vi "new FGGA Serial Data Server & Recordingv5.0_10Hz_Scroll_Pump.vi"(0 "VISA resource name out":refnum<visa-resource-name>, 11 "error IO":errorcluster) -> ()   [LabVIEW 2014]
uses:
  <vilib>/Platform/TimedLoop/XDataNode/timing_clust.ctl
  <vilib>/Platform/TimedLoop/XDataNode/nitl_modes.ctl
  <vilib>/Platform/TimedLoop/XDataNode/wakeup.ctl
  C:/Program Files (x86)/National Instruments/LabVIEW 2014/examples/Data Communication/Network Streams/Simple Network Streams/support/Network Stream Command.ctl
  <vilib>/Utility/error.llb/whitespace.ctl
  <vilib>/Instr/_visa.llb/VISA Flush IO Buffer Mask.ctl
  <vilib>/Instr/_visa.llb/VISA Configure Serial Port (Instr).vi
  <vilib>/Utility/tcp.llb/UDP Multicast Write-Only Open.vi
  <vilib>/platform/TimedLoop/XDataNode/XDataNode.xnode
  <vilib>/Platform/TimedLoop/XDataNode/XDNodeRunTimeDep.lvlib
panel:
  out "V12":bool
  out "V11":bool
  out "V10":bool
  out "FLOW ALL OFF":bool
  out "LOW FLOW MASTER SWITCH":bool
  out "HIGH FLOW MASTER SWITCH":bool
  out "ASCII_file_out":string
  out "Unix time":u32
  out "FGGA Pump":bool
  out "Flight Number":string
  out "Stop File Write":bool
  out "Default file name":string
  out "MFC":dbl[](array[numeric])
  out "FGGA restart":bool
  out "V4":bool
  out "V3":bool
  out "V2":bool
  out "V1":bool
  out "error out 2":errorcluster
  out "error out":errorcluster
  in  "MFC_1 SLPM set value":dbl
  out "Value Read":string
  out "status":bool
  in  "VISA resource name":refnum<visa-resource-name>="ASRL3::INSTR"
  in  "timeout (10sec) 2":u32=3000
  in  "Clear Display\nErrors":bool
  out "Data Processing":bool
  out "TCP Binary Packet":string
  out "UDP Time Stamp Offset":i32=1
  out "Data String":string
  out "UDP_ACSII_Out":string
  out "Serial error out":errorcluster
  out "SEPTIC TCP Error Out":errorcluster
  out "TCP packet\nSend To SEPTIC":bool
  out "FISH TCP Error Out":errorcluster
  out "TCP packet\nSend To FISH":bool
  out "UDP_Pack_num":u32
  out "UDP_Out Status":bool
  out "UDP_Out_Error Out":errorcluster
  out "Data Array":string[](array[string])
  out "RAW DATA":string
  in  "stop":bool
  out "Number of times \nRead time out":u32
  out "Loop count":i32
  # "Date"
  # "Time"
  # "CH4_wet_ppm"
  # "1"
  # "H2O_ppm"
  # "CO2_wet_ppm"
  # "CH4_dry_ppm"
  # "CO2_dry_ppm"
  # "cell_pressure_torr"
  # "cell_temp_degC"
  # "ambient(bench)_temp_degC"
  # "RDA_us"
  # "RDB_us"
  # "Fitflag"
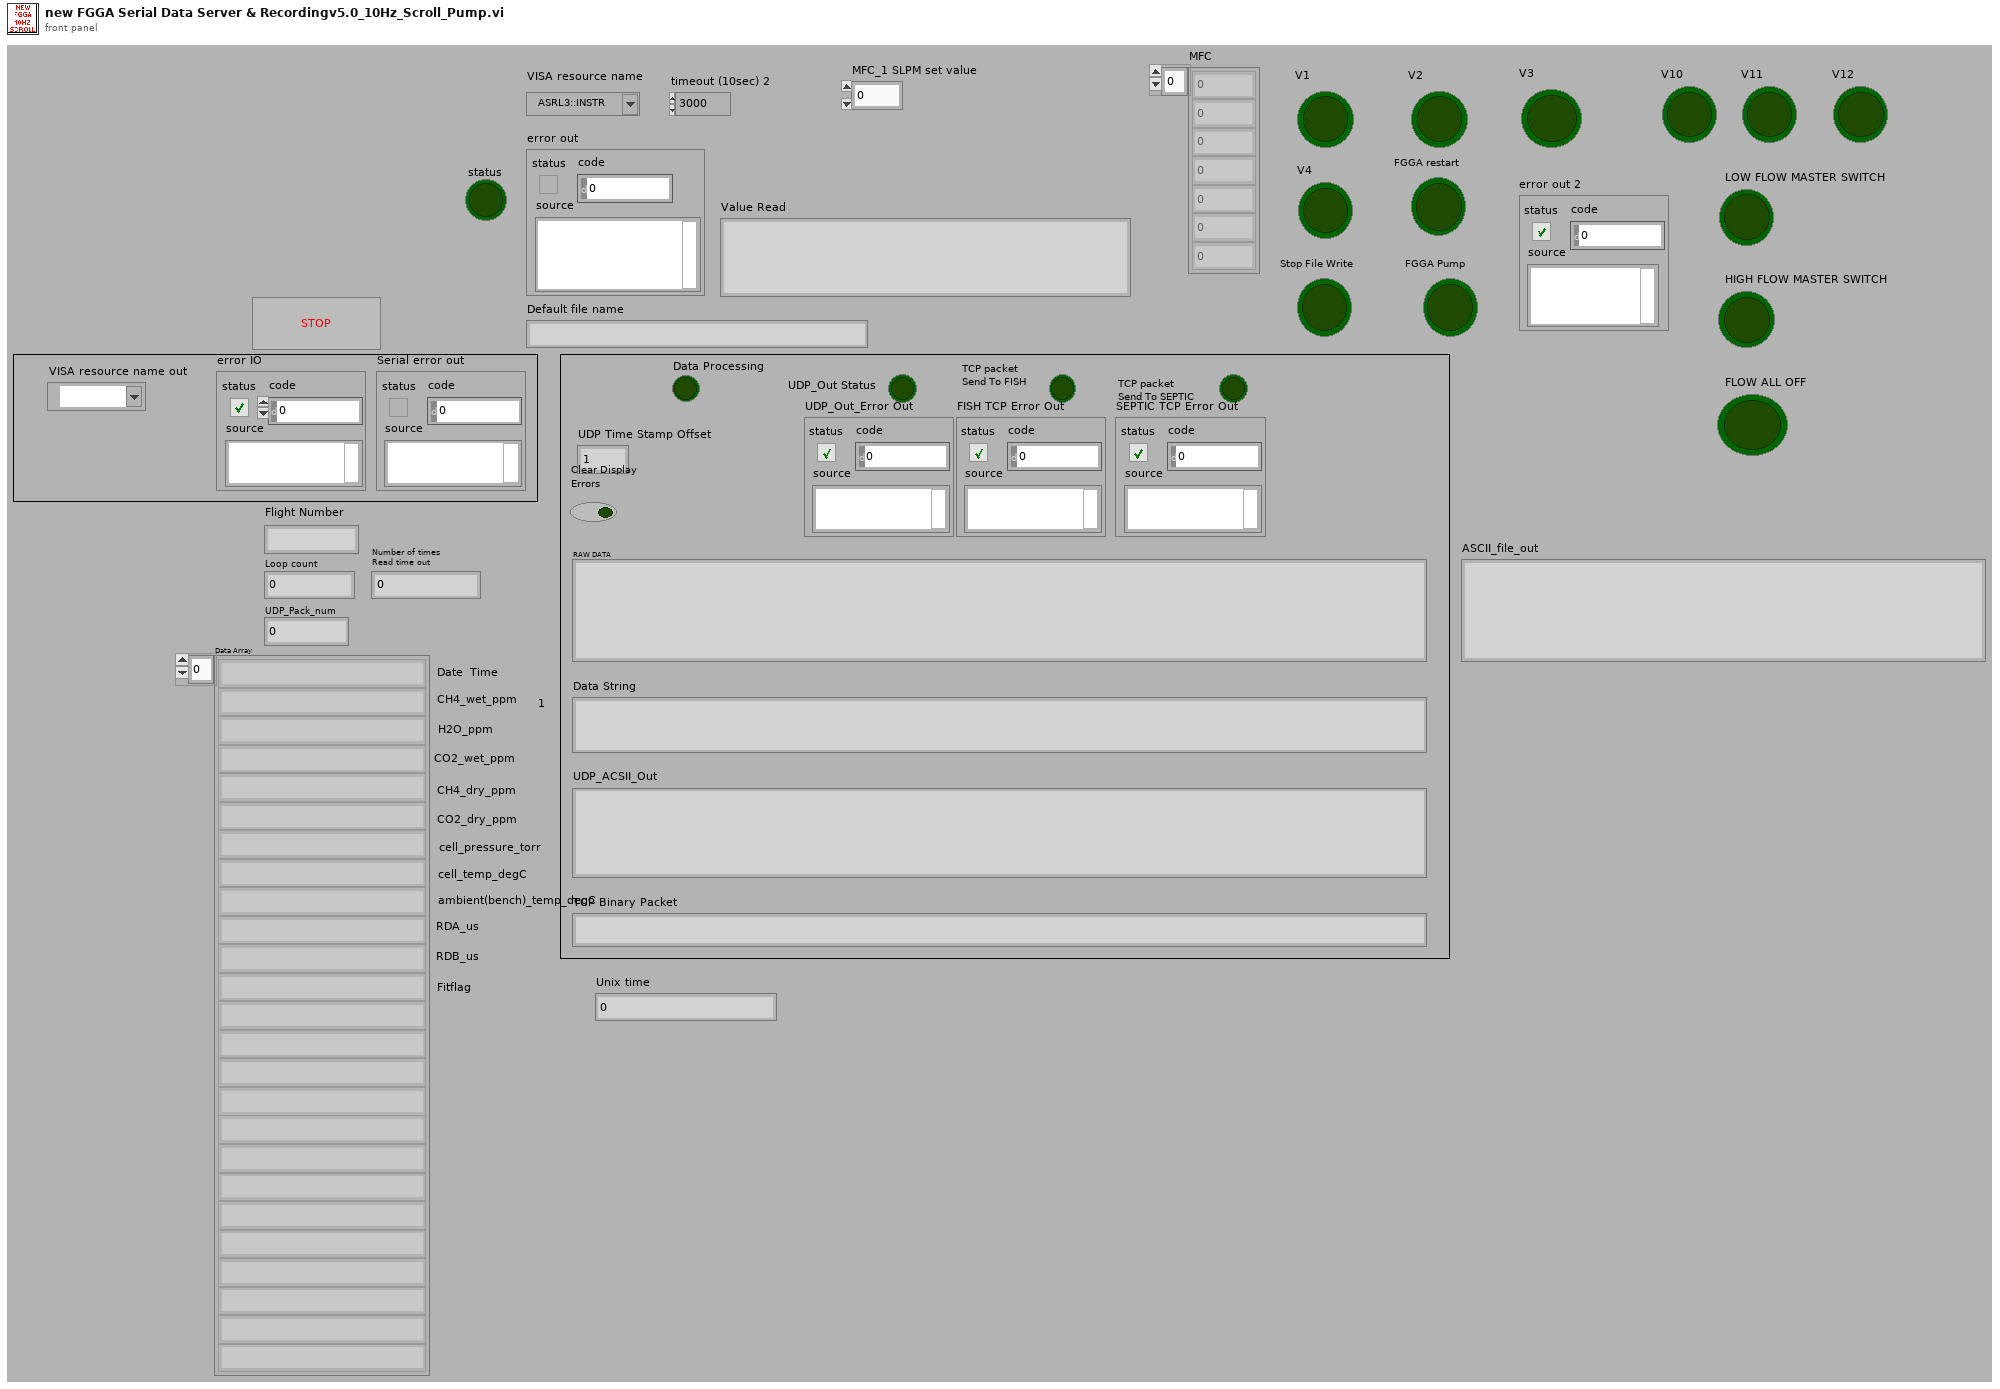
[diagram p1: front panel]
types:
  T1 = typedef "XDNodeRunTimeDep.lvlib/timing_clust.ctl" = cluster{"Expected End [f-1]":u64, "Actual End [f-1]":u64, "Finished Late? [f-1]":bool, "Expected End [i-1]":u64, "Actual End [i-1]":u64, "Finished Late? [i-1]":bool, "Expected Start [i]":u64, "Actual Start [i]":u64, "Expected Start [f]":u64, "Actual Start [f]":u64, "Source Name":string, "Structure Name":string, "Period":i64, "Deadline":i64, "Offset":i64, "Start":i64, "Priority":i32, "Timeout":i32, "Mode":T2, "Wakeup Reason":T3, "Error":errorcluster, "Source Type":string, "Secondary Source Type":string, "Global End Time":u64, "Global Start Time":u64, "Frame Duration":u64, "Iteration Duration":u64, "Assigned CPU":i32, "I/O Scan Engine Mode":u32}
  T2 = typedef "XDNodeRunTimeDep.lvlib/nitl_modes.ctl" = enum32{"No Change", "Process missed periods, maintain original phase", "Discard missed periods, maintain original phase", "Process missed periods, ignore original phase", "Discard missed periods, ignore original phase"}
  T3 = typedef "XDNodeRunTimeDep.lvlib/wakeup.ctl" = enum32{"Normal", "Aborted", "Asynchronous wakeup", "Timing source error", "Timed loop error", "Timeout"}
  T4 = enum16{"open", "replace", "create", "open or create", "replace or create", "replace or create with confirmation"}
  T5 = typedef "Network Stream Command.ctl" = cluster{"Message":string, "Message Data":variant}
  T6 = typedef "whitespace.ctl" = u16
  T7 = typedef "VISA Flush IO Buffer Mask.ctl" = u16
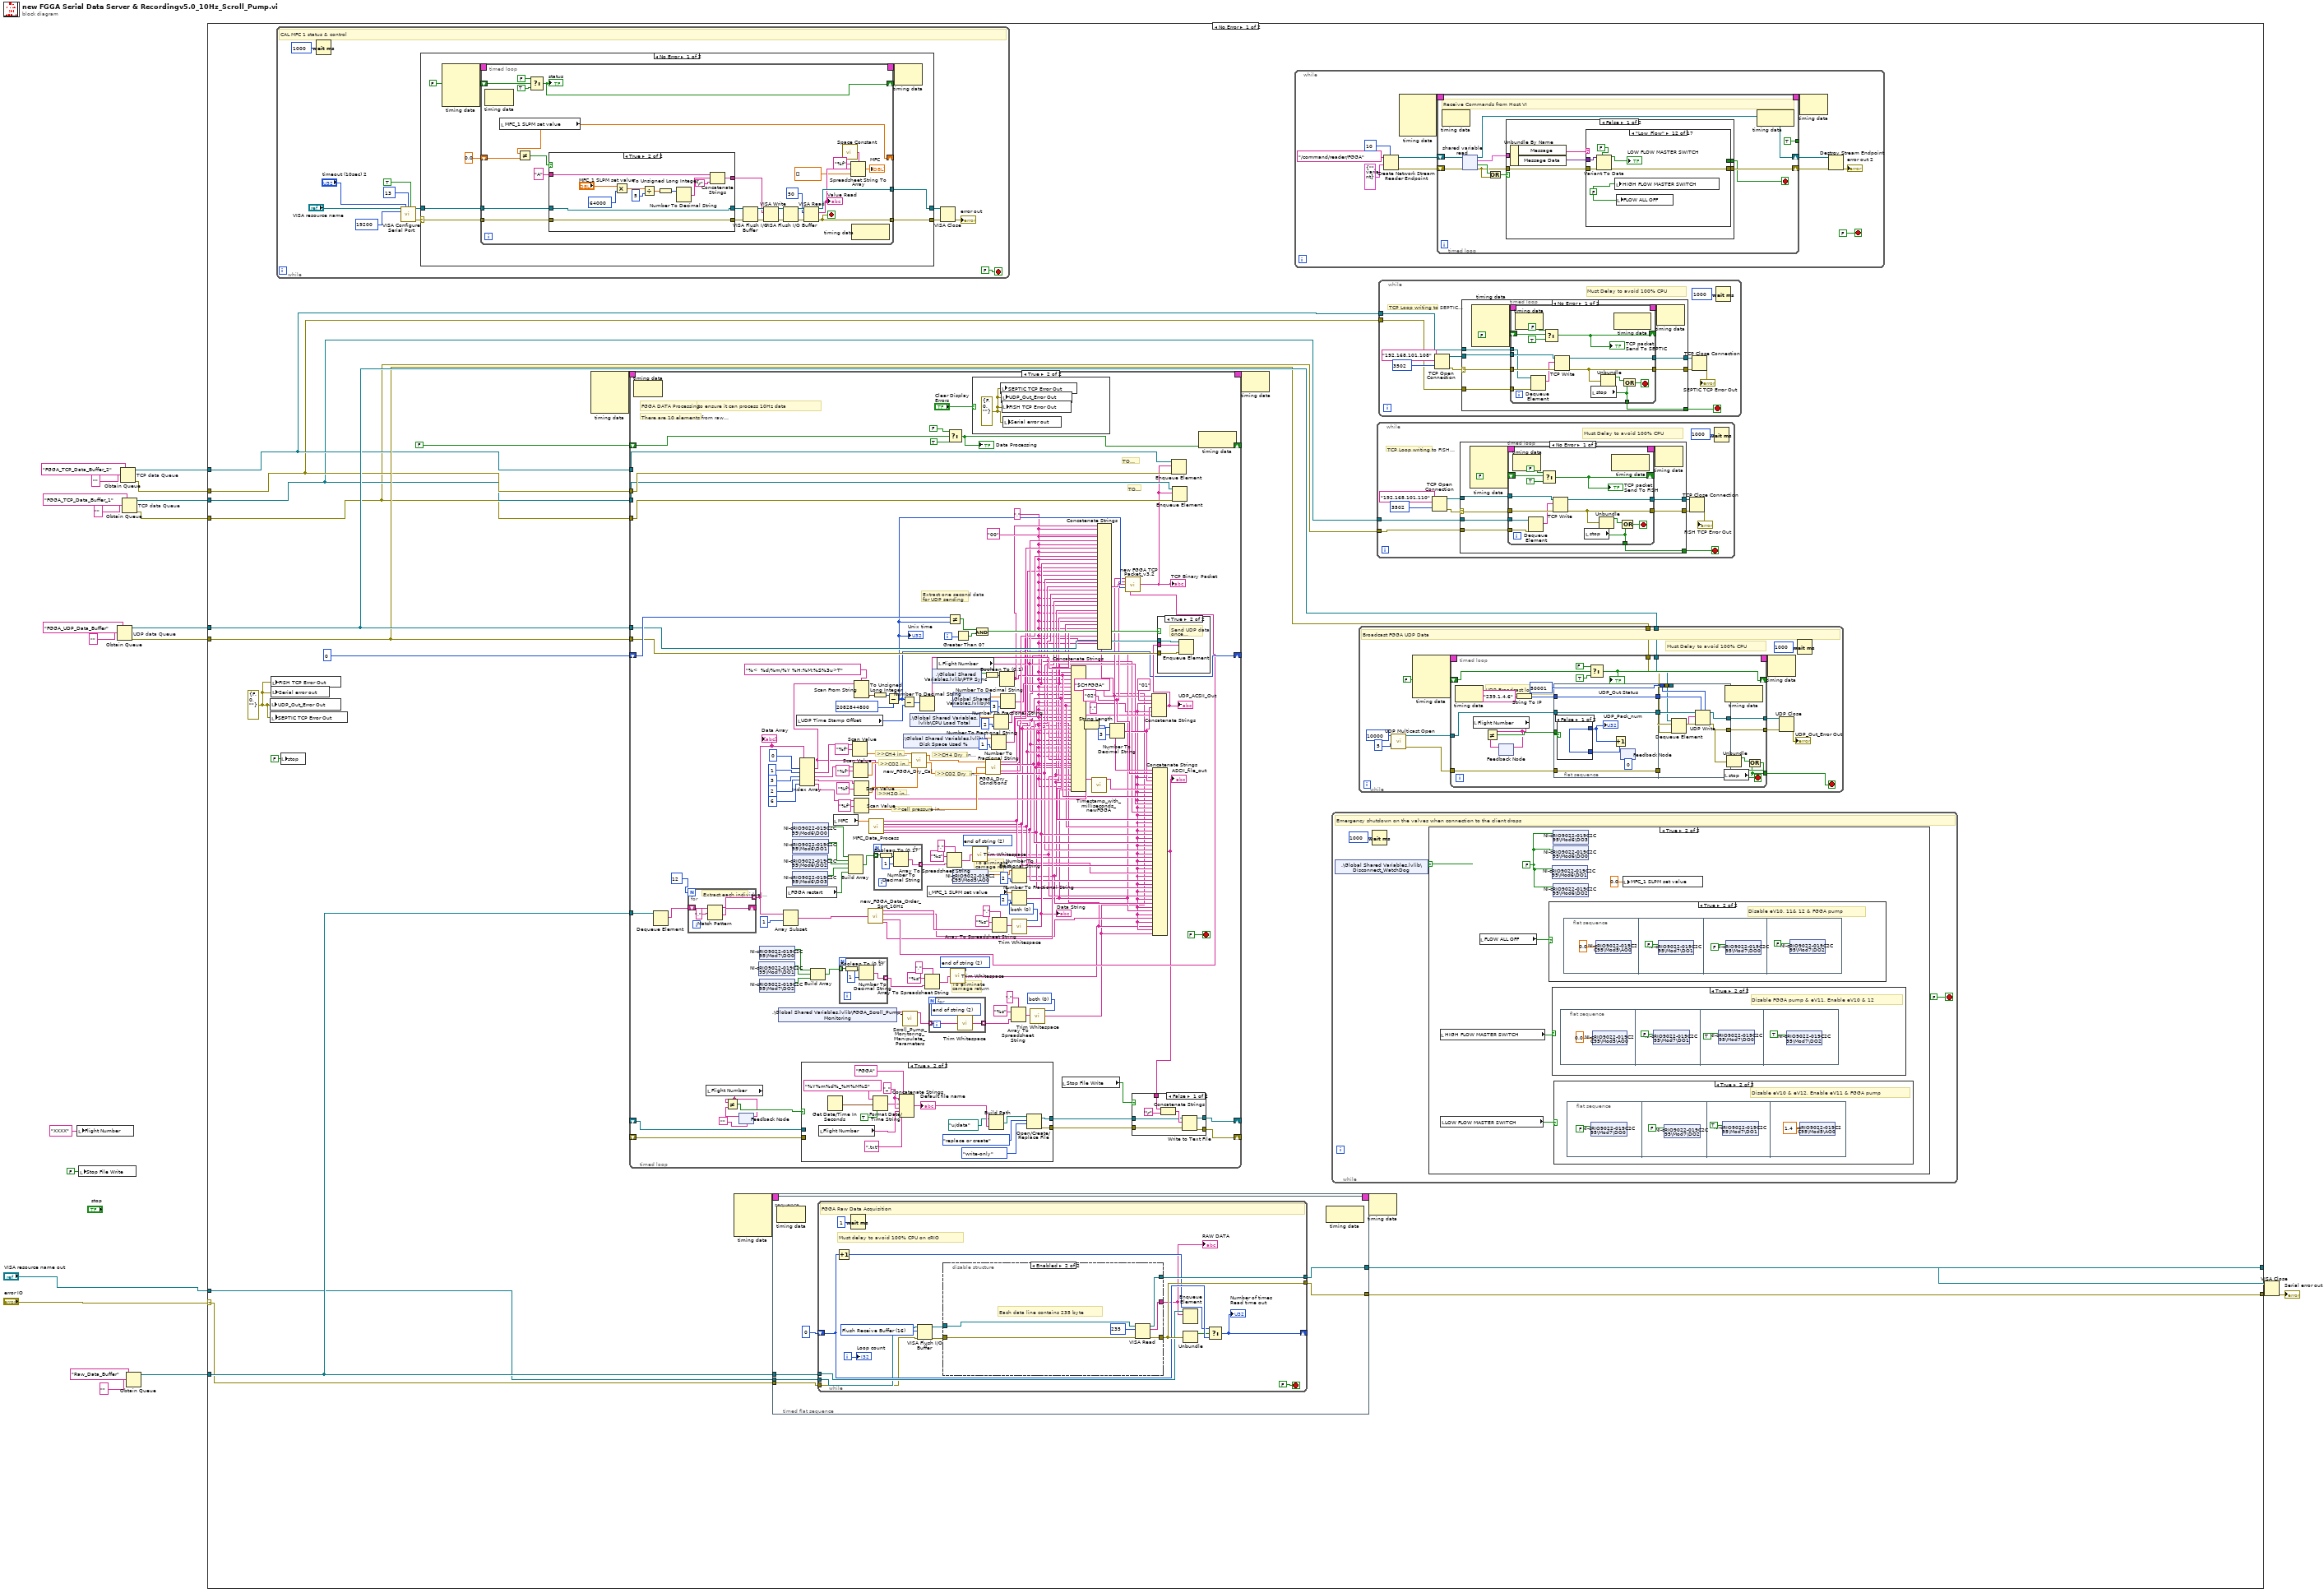
[diagram p0: block diagram]
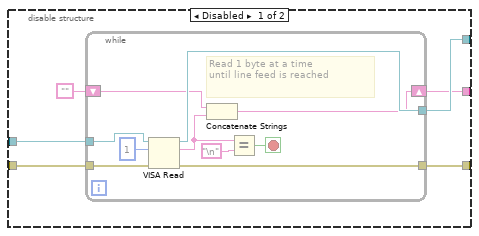
[diagram p2: hidden frame]
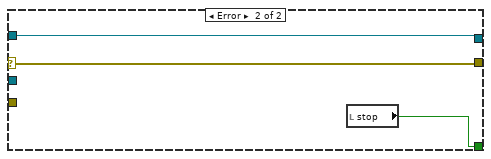
[diagram p3: hidden frame]
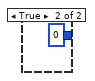
[diagram p4: hidden frame]
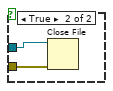
[diagram p6: hidden frame]
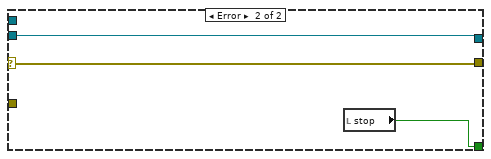
[diagram p9: hidden frame]
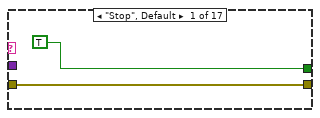
[diagram p14: hidden frame]
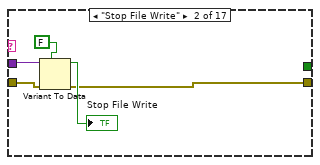
[diagram p15: hidden frame]
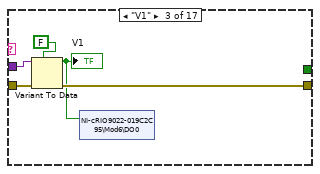
[diagram p16: hidden frame]
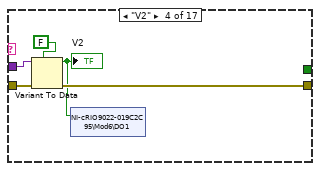
[diagram p17: hidden frame]
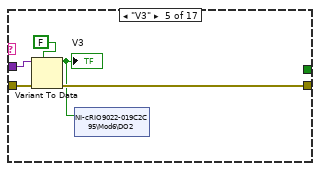
[diagram p18: hidden frame]
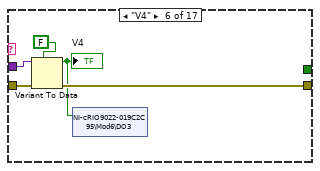
[diagram p19: hidden frame]
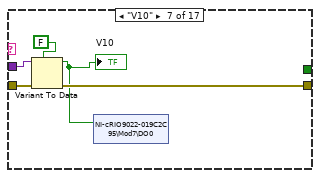
[diagram p20: hidden frame]
diagram:
  n1 = local write "Flight Number"("XXXX" ("Flight Number")) -> ()
  n2 = local write "Stop File Write"(FALSE ("Stop File Write")) -> ()
  n3 = Obtain Queue "UDP data Queue"(name (unnamed)="FGGA_UDP_Data_Buffer", element data type="") -> (queue out=w14:refnum<queue>, error out=w13:errorcluster)  [unwired: 3 in, 1 out]
  n4 = Obtain Queue "TCP data Queue"(name (unnamed)="FGGA_TCP_Data_Buffer_2", element data type="") -> (queue out=w8:refnum<queue>, error out=w7:errorcluster)  [unwired: 3 in, 1 out]
  n5 = Obtain Queue "TCP data Queue"(name (unnamed)="FGGA_TCP_Data_Buffer_1", element data type="") -> (queue out=w6:refnum<queue>, error out=w5:errorcluster)  [unwired: 3 in, 1 out]
  n6 = Obtain Queue(name (unnamed)="Raw_Data_Buffer", element data type="") -> (queue out=w20:refnum<queue>)  [unwired: 3 in, 2 out]
  n7 = case shown="No Error" "error IO" {
    selector: "error IO" -> [w28 w643]
    tunnel: "VISA resource name out" -> [w29 w644]
    tunnel: [w40 w644] -> w17
    tunnel: [w41 w643] -> w18
    tunnel: w20 -> [w39 _]
    tunnel: w14 -> [w37 _]
    tunnel: w13 -> [w36 _]
    tunnel: w8 -> [w35 _]
    tunnel: w7 -> [w34 _]
    tunnel: w6 -> [w33 _]
    tunnel: w5 -> [w32 _]
    frame No Error {
      w25 = errorcluster {"status"=FALSE, "code"=0, "source"=""} ("UDP Error Out")
      n8 = local write "UDP_Out_Error Out"(w25) -> ()
      n9 = local write "SEPTIC TCP Error Out"(w25) -> ()
      n10 = local write "FISH TCP Error Out"(w25) -> ()
      n11 = local write "Serial error out"(w25) -> ()
      n12 = while {
        stop <- FALSE stop-if-true
        # "CAL MFC 1 status & control"
        n13 = Wait (ms)(milliseconds to wait=u32 1000) -> ()  [unwired: 1 out]
        n14 = call-poly "VISA Configure Serial Port"("VISA resource name"="VISA resource name", "timeout (10sec)"="timeout (10sec) 2", "termination char\n(0xA = '\\n' = LF)"=u8 13 ("termination char\n(0xA = '\\n' = LF)"), "Enable Termination\nChar (T)"=TRUE ("Enable Termination\nChar (T)"), "baud rate (9600)"=u32 19200) -> ("VISA resource name out"=w584:refnum<visa-resource-name>, "error out"=w580:errorcluster)  [unwired: 9 in]
        n15 = case shown="No Error" w580 {
          selector: w580 -> [w591 w641]
          tunnel: w584 -> [w592 w642]
          tunnel: [w590 w642] -> w583
          tunnel: [w589 w641] -> w582
          frame No Error {
            n16 = node-c288() -> (w587:T1)  [unwired: 4 in]
            n17 = timed-loop {
              tunnel: w592 -> [w615]
              tunnel: w591 -> [w613]
              tunnel: [w606] -> w590
              tunnel: [w601] -> w589
              shift-right: [w602] -> _
              shift-left: FALSE -> [w605]
              timing: w587 -> [_]
              timing-out: [_] -> w586
              shift-right: [w593] -> _
              shift-left: 0.0 -> [w595]
              stop <- w601 stop-if-true
              n18 = node-c288() -> ()  [unwired: 1 in, 1 out]
              n19 = local read "MFC_1 SLPM set value"() -> (w593:dbl)
              n20 = Not Equal?(x=w593, y=w595) -> (x != y?=w594:bool)
              n21 = Select(t=FALSE, s=w605, f=TRUE) -> (s? t:f=w602:bool)
              "status" <- w602
              n22 = case shown="True" w594 {
                tunnel: w615 -> [w623 w638]
                tunnel: [w623 w638] -> w614
                tunnel: w613 -> [w622 w637]
                tunnel: [w622 w637] -> w612
                tunnel: "A" -> [w626 w630]
                tunnel: [w624 w627] -> w610
                frame False {
                  n23 = Concatenate Strings(w626, "\r") -> (w624:string)
                }
                frame True {
                  n24 = Multiply(x="MFC_1 SLPM set value", y=u32 64000) -> (x*y=w634:dbl)
                  n25 = Divide(x=w634, y=u32 5) -> (x/y=w632:dbl)
                  n26 = To Unsigned Long Integer(number=w632) -> (unsigned 32bit integer=w631:u32)
                  n27 = Number To Decimal String(number=w631) -> (decimal integer string=w629:string)  [unwired: 1 in]
                  n28 = Concatenate Strings(w630, w629, "\r") -> (w627:string)
                }
              }
              n29 = VISA Flush I/O Buffer(VISA resource name=w614, error in (no error)=w612) -> (VISA resource name out=w617:refnum<visa-resource-name>, error out=w616:errorcluster)  [unwired: 1 in]
              n30 = VISA Write(VISA resource name=w617, write buffer=w610, error in (no error)=w616) -> (VISA resource name out=w609:refnum<visa-resource-name>, error out=w608:errorcluster)  [unwired: 1 out]
              n31 = VISA Flush I/O Buffer(VISA resource name=w609, error in (no error)=w608) -> (VISA resource name out=w619:refnum<visa-resource-name>, error out=w618:errorcluster)  [unwired: 1 in]
              n32 = VISA Read(VISA resource name=w619, byte count=u32 50, error in (no error)=w618) -> (VISA resource name out=w606:refnum<visa-resource-name>, read buffer=w600:string, error out=w601:errorcluster)  [unwired: 1 out]
              "Value Read" <- w600
              n33 = call <vilib>:"Space Constant.vi"() -> ("String"=w599:string)
              n34 = Spreadsheet String To Array(delimiter (Tab)=w599, format string="%f", spreadsheet string=w600, array type (2D Dbl)=dbl[] []) -> (array=→"MFC":dbl[])
              n35 = node-c288() -> ()  [unwired: 1 in, 1 out]
            }
            n36 = node-c288(w586) -> ()  [unwired: 1 out]
          }
          frame Error {
          }
        }
        n37 = VISA Close(VISA resource name=w583, error in (no error)=w582) -> (error out=→"error out":errorcluster)
      }
      n38 = local write "stop"(FALSE ("stop")) -> ()
      n39 = node-c288() -> (w27:T1)  [unwired: 4 in]
      n40 = timed-loop {
        timing: w27 -> [_]
        timing-out: [_] -> w26
        tunnel: w39 -> [w340]
        tunnel: w37 -> [w309]
        tunnel: w36 -> [w308]
        shift-right: [w251] -> _
        shift-left: u32 0 -> [w312]
        tunnel: w35 -> [w307]
        tunnel: w34 -> [w306]
        tunnel: w33 -> [w305]
        tunnel: w32 -> [w304]
        shift-right: [w300] -> _
        shift-left: FALSE -> [w303]
        shift-right: [w291] -> _
        shift-left: _ -> [w283]
        shift-right: [w281] -> _
        shift-left: _ -> [w282]
        i -> [w311]
        stop <- FALSE stop-if-true
        w202 = T6 0 items=["both", "start of string", "end of string"] ("location (both)")
        w207 = T6 2 items=["both", "start of string", "end of string"] ("location (both)")
        w257 = T6 2 items=["both", "start of string", "end of string"] ("location (both)")
        w198 = ","
        w329 = T6 0 items=["both", "start of string", "end of string"] ("location (both)")
        w215 = ","
        w238 = "02"
        w239 = "$CHFGGA"
        # "To eliminate\ncarriage return"
        # "To eliminate\ncarriage return"
        # ">>cell pressure in torr>>"
        # "There are 10 elements from raw packet"
        # "TO SEPTIC"
        # "TO FISH"
        # "Extract one second data\nfor UDP sending"
        # ">>CO2 Dry  in ppm>>"
        # ">>CH4 Dry  in ppb>>"
        # ">>H2O in ppm>>"
        # ">>CO2 in ppm>>"
        # ">>CH4 in ppm>>"
        # "Loop Time is 50msec to ensure it can process 10Hz data"
        # "FGGA DATA Processing"
        n41 = node-c288() -> ()  [unwired: 1 in, 1 out]
        n42 = Dequeue Element(queue=w340) -> (element=w299:string)  [unwired: 2 in, 3 out]
        n43 = for {
          N: 12 -> [_]
          shift-right: [w384] -> _
          shift-left: w299 -> [w382]
          tunnel: [w383] -> w334 mode=indexing
          # "Extract each individual param"
          n44 = Match Pattern(string=w382, regular expression=",") -> (before substring=w383:string, after substring=w384:string)  [unwired: 1 in, 2 out]
        }
        "Data Array" <- w334
        n45 = local read "Flight Number"() -> (w280:string)
        n46 = feedback #1("" ("Flight Number")) -> (w288:string)
        n47 = Not Equal?(x=w280, y=w288) -> (x != y?=w286:bool)
        n48 = feedback-in #1(w280) -> ()
        n49 = shared-variable "NI-cRIO9022-019C2C95\\Mod7\\DO1"() -> (w212:bool)  [unwired: 1 in, 1 out]
        n50 = shared-variable "NI-cRIO9022-019C2C95\\Mod7\\DO0"() -> (w213:bool)  [unwired: 1 in, 1 out]
        n51 = shared-variable "NI-cRIO9022-019C2C95\\Mod7\\DO2"() -> (w211:bool)  [unwired: 1 in, 1 out]
        n52 = shared-variable ".\\Global Shared Variables.lvlib\\FGGA_Scroll_Pump_Monitoring"() -> (w200:string[])  [unwired: 1 in, 1 out]
        n53 = Array Subset(array=w334, index=1) -> (w244:string[])  [unwired: 1 in]
        n54 = local read "FGGA restart"() -> (w265:bool)
        n55 = shared-variable "NI-cRIO9022-019C2C95\\Mod6\\DO2"() -> (w271:bool)  [unwired: 1 in, 1 out]
        n56 = shared-variable "NI-cRIO9022-019C2C95\\Mod6\\DO3"() -> (w270:bool)  [unwired: 1 in, 1 out]
        n57 = shared-variable "NI-cRIO9022-019C2C95\\Mod6\\DO0"() -> (w273:bool)  [unwired: 1 in, 1 out]
        n58 = shared-variable "NI-cRIO9022-019C2C95\\Mod6\\DO1"() -> (w272:bool)  [unwired: 1 in, 1 out]
        n59 = local read "UDP Time Stamp Offset"() -> (w256:i32)
        n60 = Index Array(array=w334, index #1=0 ("index"), index #2=1 ("index"), index #3=3 ("index"), index #4=2 ("index"), index #5=6 ("index")) -> (element #1=w234:string, element #2=w250:string, element #3=w249:string, element #4=w248:string, element #5=w247:string)
        n61 = case shown="True" w286 {
          tunnel: [w353 w355] -> w285
          tunnel: [w352 w354] -> w284
          tunnel: w283 -> [w353 _]
          tunnel: w282 -> [w352 _]
          frame False {
          }
          frame True {
            w361 = "_" ("string")
            n62 = local read "Flight Number"() -> (w368:string)
            n63 = Get Date/Time In Seconds() -> (seconds since 1Jan1904=w356:timestamp)
            n64 = Format Date/Time String(time format string (%c)="%Y%m%d%_%H%M%S", seconds (now)=w356, UTC format=TRUE) -> (date/time string=w358:string)
            n65 = Concatenate Strings("FGGA" ("string"), w361, w358, w361, w368, ".txt" ("string")) -> (w363:string)
            "Default file name" <- w363
            n66 = Build Path(base path=path "u:/data", name or relative path=w363) -> (appended path=w367:path)
            n67 = Open/Create/Replace File(file path (use dialog)=w367, operation (0:open)=T4."replace or create", access (0:read/write)=enum16{"read/write", "read-only", "write-only"}."write-only") -> (refnum out=w355:refnum<file>, error out=w354:errorcluster)  [unwired: 3 in, 1 out]
          }
        }
        n68 = Build Array(w213, w212, w211) -> (w214:bool[])
        n69 = local read "MFC"() -> (w292:dbl[])
        n70 = for {
          tunnel: w214 -> [w346] mode=indexing
          tunnel: [w345] -> w206 mode=indexing
          n71 = Boolean To (0,1)(Boolean=w346) -> (0, 1=w347:i16)
          n72 = Number To Decimal String(number=w347, width (-)=i16 1) -> (decimal integer string=w345:string)
        }
        n73 = Build Array(w273, w272, w271, w270, w265) -> (w269:bool[])
        n74 = Scan Value(string=w250, format string="%f") -> (value=w321:dbl)  [unwired: 1 in, 1 out]
        n75 = Scan Value(string=w249, format string="%f") -> (value=w320:dbl)  [unwired: 1 in, 1 out]
        n76 = Scan From String(format string="%<  %d/%m/%Y %H:%M:%S%3u>T", input string=w234) -> (output 1=w317:timestamp)  [unwired: 3 in, 3 out]
        n77 = Scan Value(string=w248, format string="%f") -> (value=w293:dbl)  [unwired: 1 in, 1 out]
        n78 = Scan Value(string=w247, format string="%f") -> (value=w294:dbl)  [unwired: 1 in, 1 out]
        n79 = call "new_FGGA_Data_Order_Sort_10Hz.vi"("Data In"=w244) -> ("UDP Data Out"=w243:string[], "ASCII Ambient(bench)_temp"=w216:string, "TCP Data Out"=w242:string[], "TCP Ambient(bench)_temp"=w241:string)  [unwired: 11 in]
        n80 = call "MFC_Data_Process.vi"("MFC"=w292) -> ("MFC Absolute Pressure"=w224:string, "MFC Temperature"=w223:string, "MFC Volumetric Flow"=w222:string, "MFC Mass Flow"=w221:string, "MFC Set Point"=w220:string)  [unwired: 10 in]
        n81 = To Unsigned Long Integer(number=w317) -> (unsigned 32bit integer=w318:u32)
        n82 = for {
          tunnel: w269 -> [w350] mode=indexing
          tunnel: [w349] -> w266 mode=indexing
          n83 = Boolean To (0,1)(Boolean=w350) -> (0, 1=w351:i16)
          n84 = Number To Decimal String(number=w351, width (-)=i16 1) -> (decimal integer string=w349:string)
        }
        n85 = Subtract(x=w318, y=u32 2082844800) -> (x-y=w251:u32)
        "Unix time" <- w251
        n86 = Subtract(x=w251, y=w256) -> (x-y=w315:u32)
        n87 = call "Scroll_Pump_Monitoring_Manipulate_Parameters.vi"("FGGA_Scroll_Pump\nMonitoring_Input"=w200) -> ("output array"=w199:string[])  [unwired: 14 in]
        n88 = shared-variable ".\\Global Shared Variables.lvlib\\Disk Space Used %"() -> (w259:dbl)  [unwired: 1 in, 1 out]
        n89 = shared-variable ".\\Global Shared Variables.lvlib\\CPU Load Total"() -> (w279:dbl)  [unwired: 1 in, 1 out]
        n90 = call "new_FGGA_Dry_Cal.vi"("H2O"=w293, "CO2_Wet"=w320, "CH4_Wet"=w321) -> ("CO2_Dry"=w296:dbl, "CH4_Dry"=w298:dbl)  [unwired: 7 in]
        n91 = Number To Decimal String(number=w315) -> (decimal integer string=w316:string)  [unwired: 1 in]
        n92 = Array To Spreadsheet String(delimiter (Tab)=",", array=w206, 3:"%s" ("format string")) -> (spreadsheet string=w208:string)
        n93 = local read "MFC_1 SLPM set value"() -> (w261:dbl)
        n94 = for {
          tunnel: w199 -> [w343] mode=indexing
          tunnel: [w342] -> w201 mode=indexing
          w341 = T6 2 items=["both", "start of string", "end of string"] ("location (both)")
          n95 = call <vilib>:"Trim Whitespace.vi"("string"=w343, "location (both)"=w341) -> ("trimmed string"=w342:string)
        }
        n96 = shared-variable ".\\Global Shared Variables.lvlib\\PTP Sync"() -> (w274:bool)  [unwired: 1 in, 1 out]
        n97 = local read "Flight Number"() -> (w230:string)
        n98 = Array To Spreadsheet String(delimiter (Tab)=",", array=w266, 3:"%s" ("format string")) -> (spreadsheet string=w258:string)
        n99 = Select(t=FALSE, s=w303, f=TRUE) -> (s? t:f=w300:bool)
        "Data Processing" <- w300
        n100 = Not Equal?(x=w312, y=w251) -> (x != y?=w313:bool)
        n101 = call <vilib>:"Trim Whitespace.vi"("string"=w208, "location (both)"=w207) -> ("trimmed string"=w197:string)
        n102 = shared-variable ".\\Global Shared Variables.lvlib\\MFM"() -> (w277:dbl)  [unwired: 1 in, 1 out]
        n103 = shared-variable "NI-cRIO9022-019C2C95\\Mod5\\AO0"() -> (w263:dbl)  [unwired: 1 in, 1 out]
        n104 = Greater Than 0?(x=w311) -> (x > 0?=w314:bool)
        n105 = case shown="True" "Clear Display\nErrors" {
          frame False {
          }
          frame True {
            w378 = errorcluster {"status"=FALSE, "code"=0, "source"=""} ("UDP Error Out")
            n106 = local write "SEPTIC TCP Error Out"(w378) -> ()
            n107 = local write "UDP_Out_Error Out"(w378) -> ()
            n108 = local write "FISH TCP Error Out"(w378) -> ()
            n109 = local write "Serial error out"(w378) -> ()
          }
        }
        n110 = call <vilib>:"Trim Whitespace.vi"("string"=w258, "location (both)"=w257) -> ("trimmed string"=w219:string)
        n111 = Compound Arithmetic op=AND(w313, w314) -> (w310:bool)
        n112 = Boolean To (0,1)(Boolean=w274) -> (0, 1=w275:i16)
        n113 = call "FGGA_Dry_Conditions.vi"("CH4_Dry"=w298, "Pressure"=w294, "CO2_Dry"=w296) -> ("CH4_Dry_TCP"=w255:string, "CH4_Dry_UDP"=w226:string, "CO2_Dry_TCP"=w254:string, "CO2_Dry_UDP"=w225:string)  [unwired: 9 in]
        n114 = Number To Fractional String(number=w259, precision (6)=i16 1) -> (F-format string=w228:string)  [unwired: 2 in]
        n115 = Array To Spreadsheet String(delimiter (Tab)=",", array=w243, 3:"%s" ("format string")) -> (spreadsheet string=w328:string)
        n116 = Number To Fractional String(number=w279, precision (6)=i16 2) -> (F-format string=w229:string)  [unwired: 2 in]
        n117 = Number To Decimal String(number=w275) -> (decimal integer string=w232:string)  [unwired: 1 in]
        n118 = Number To Fractional String(number=w277, precision (6)=i16 3) -> (F-format string=w231:string)  [unwired: 2 in]
        n119 = Array To Spreadsheet String(delimiter (Tab)=",", array=w201, 3:"%s" ("format string")) -> (spreadsheet string=w203:string)
        n120 = Number To Fractional String(number=w263, precision (6)=i16 2) -> (F-format string=w218:string)  [unwired: 2 in]
        n121 = Number To Fractional String(number=w261, precision (6)=i16 2) -> (F-format string=w217:string)  [unwired: 2 in]
        n122 = call <vilib>:"Trim Whitespace.vi"("string"=w328, "location (both)"=w329) -> ("trimmed string"=w227:string)
        "Data String" <- w227
        n123 = call <vilib>:"Trim Whitespace.vi"("string"=w203, "location (both)"=w202) -> ("trimmed string"=w196:string)
        n124 = local read "Stop File Write"() -> (w289:bool)
        n125 = Concatenate Strings(w316, w198, w232, w198, w231, w198, w230, w198, w229, w198, w228, w198, w227, w198, w226, w198, w225, w198, w224, w198, w223, w198, w222, w198, w221, w198, w220, w198, w219, w198, w218, w198, w217) -> (w236:string)
        n126 = String Length(string=w236) -> (length=w337:i32)
        n127 = call "Timestamp_with_milliseconds_newFGGA.vi"("Input Time"=w234) -> ("Output Time"=w233:string)  [unwired: 14 in]
        n128 = Concatenate Strings(w232, w198, "00", w198, w230, w198, w255, w198, w254, w198, w231, w198, w224, w198, w223, w198, w222, w198, w221, w198, w220, w198, w219, w198, w218, w198, w217, w198, w241, w198, w197, w198, w196) -> (w253:string)
        n129 = Number To Decimal String(number=w337, width (-)=i16 3) -> (decimal integer string=w237:string)
        n130 = call "new FGGA TCP Packet_v3.2.vi"("ID"=w239, "Version"=w238, "TCP Packet In"=w253, "utc_time"=w251, "Data Array"=w242) -> ("TCP Binary Packet"=w245:string)  [unwired: 10 in]
        "TCP Binary Packet" <- w245
        n131 = Concatenate Strings(w239, "01", w215, w237, w215, w236) -> (w290:string)
        "UDP_ACSII_Out" <- w290
        n132 = Concatenate Strings(w239, w238, w215, w237, w215, w233, w215, w232, w215, w231, w215, w230, w215, w229, w215, w228, w215, w227, w215, w226, w215, w225, w215, w224, w215, w223, w215, w222, w215, w221, w215, w220, w215, w219, w215, w218, w215, w217, w215, w216, w215, w197, w215, w196) -> (w235:string)
        "ASCII_file_out" <- w235
        n133 = case shown="False" w289 {
          tunnel: w235 -> [w375 _]
          tunnel: [w372 _] -> w291
          tunnel: w285 -> [w371 w377]
          tunnel: w284 -> [w370 w376]
          tunnel: [w369 _] -> w281
          frame False {
            n134 = Concatenate Strings(w375, "\r") -> (w373:string)
            n135 = Write to Text File(file (use dialog)=w371, text=w373, error in=w370) -> (refnum out=w372:refnum<file>, error out=w369:errorcluster)  [unwired: 2 out]
          }
          frame True {
            n136 = Close File(refnum=w377, error in=w376) -> ()  [unwired: 2 out]
          }
        }
        n137 = case shown="True" w310 {
          tunnel: w290 -> [_ w381]
          tunnel: w309 -> [_ w380]
          tunnel: w308 -> [_ w379]
          frame False {
          }
          frame True {
            # "Send UDP data once\na second"
            n138 = Enqueue Element(queue=w380, element=w381, error in (no error)=w379) -> ()  [unwired: 1 in, 3 out]
          }
        }
        n139 = Enqueue Element(queue=w307, element=w245, error in (no error)=w306) -> ()  [unwired: 1 in, 3 out]
        n140 = Enqueue Element(queue=w305, element=w245, error in (no error)=w304) -> ()  [unwired: 1 in, 3 out]
        n141 = node-c288() -> ()  [unwired: 1 in, 1 out]
      }
      n142 = node-c288() -> (w24:T1)  [unwired: 4 in]
      n143 = timed-sequence {
        timing: w24 -> [_]
        timing-out: [_] -> w23
        tunnel: [w46] -> w41
        tunnel: [w45] -> w40
        tunnel: w39 -> [w44]
        tunnel: w29 -> [w43]
        tunnel: w28 -> [w42]
        n144 = timed-flat-sequence {
          tunnel: [w52] -> w46
          tunnel: [w51] -> w45
          tunnel: w44 -> [w50]
          tunnel: w43 -> [w49]
          tunnel: w42 -> [w48]
          n145 = node-c288() -> ()  [unwired: 1 in, 1 out]
          n146 = while {
            tunnel: w49 -> [w59]
            tunnel: w48 -> [w58]
            tunnel: [w70] -> w52
            shift-right: [w66] -> _
            shift-left: u32 0 -> [w67]
            tunnel: [w69] -> w51
            tunnel: w50 -> [w64]
            i -> [w68]
            stop <- FALSE stop-if-true
            w55 = T7 16 items=["Flush Receive Buffer"=16, "Write Transmit Buffer to Device"=32, "Flush Receive Buffer (No I/O)"=64, "Flush Transmit Buffer"=128] ("Mask")
            # "Must delay to avoid 100% CPU on cRIO"
            # "FGGA Raw Data Acquisition"
            n147 = Increment(x=w67) -> (x+1=w65:u32)
            n148 = Wait (ms)(milliseconds to wait=u32 1) -> ()  [unwired: 1 out]
            n149 = VISA Flush I/O Buffer(VISA resource name=w59, mask (16)=w55, error in (no error)=w58) -> (VISA resource name out=w56:refnum<visa-resource-name>, error out=w57:errorcluster)
            n150 = disable-structure shown="Enabled" {
              disable-tunnel: [w76 w90] -> w70
              disable-tunnel: [w75 w89] -> w69
              disable-tunnel: [w74 w88] -> w61
              disable-tunnel: w57 -> [w73 w91]
              disable-tunnel: w56 -> [w72 w92]
              frame Disabled {
                n151 = while {
                  tunnel: [w86] -> w75
                  tunnel: [w85] -> w76
                  tunnel: w72 -> [w84]
                  tunnel: w73 -> [w83]
                  shift-right: [w81] -> w74
                  shift-left: "" -> [w82]
                  stop <- w78 stop-if-true
                  # "Read 1 byte at a time \nuntil line feed is reached"
                  n152 = VISA Read(VISA resource name=w84, byte count=u32 1, error in (no error)=w83) -> (VISA resource name out=w86:refnum<visa-resource-name>, read buffer=w80:string, error out=w85:errorcluster)  [unwired: 1 out]
                  n153 = Concatenate Strings(w82, w80) -> (w81:string)
                  n154 = Equal?(x=w80, y="\n") -> (x = y?=w78:bool)
                }
              }
              frame Enabled {
                # "Each data line contains 235 byte"
                n155 = VISA Read(VISA resource name=w92, byte count=u32 235, error in (no error)=w91) -> (VISA resource name out=w89:refnum<visa-resource-name>, read buffer=w88:string, error out=w90:errorcluster)  [unwired: 1 out]
              }
            }
            "RAW DATA" <- w61
            n156 = Enqueue Element(queue=w64, element=w61) -> ()  [unwired: 2 in, 3 out]
            n157 = Unbundle(w70) -> ("status"=w63:bool)  [unwired: 2 out]
            n158 = Select(t=w65, s=w63, f=w67) -> (s? t:f=w66:u32)
            "Number of times \nRead time out" <- w66
            "Loop count" <- w68
          }
          n159 = node-c288() -> ()  [unwired: 1 in, 1 out]
        }
      }
      n160 = node-c288(w26) -> ()  [unwired: 1 out]
      n161 = while {
        stop <- FALSE stop-if-true
        n162 = Create Network Stream Reader Endpoint(7:10 ("reader buffer size"), 9:T5 {"Message"="", "Message Data"=variant} ("Message Cluster"), 11:"/command/reader/FGGA" ("reader url")) -> (0:w458:errorcluster, 3:w459:refnum<k21>)  [unwired: 4 in]
        n163 = node-c288() -> (w453:T1)  [unwired: 4 in]
        n164 = timed-loop "Host->Target Command Reader" {
          shift-right: [w469] -> w456
          shift-left: w458 -> [w472]
          shift-right: [w470] -> w455
          shift-left: w459 -> [w471]
          tunnel: [TRUE] -> _
          timing: w453 -> [_]
          timing-out: [_] -> w452
          stop <- w463 stop-if-true
          # "Receive Commands from Host VI"
          n165 = node-c288() -> ()  [unwired: 1 in, 1 out]
          n166 = shared-variable-read(w471, w472) -> (w470:refnum<k21>, w465:errorcluster, w467:bool, w468:T5)  [unwired: 1 in]
          n167 = Or(x=w467, y=w465) -> (x .or. y?=w466:bool)
          n168 = case shown="False" w466 {
            selector: w466 -> [_ w569]
            tunnel: w465 -> [w480 w570]
            tunnel: [w479 w570] -> w469
            tunnel: w468 -> [w477 _]
            tunnel: [w478 w569] -> w463
            frame False {
              n169 = Unbundle By Name(w477) -> ("Message"=w476:string, "Message Data"=w475:variant)
              n170 = case shown="\"Low_Flow\"" w476 {
                tunnel: w480 -> [w482 w487 w492 w497 w502 w507 w512 w517 w522 w528 w534 w540 w545 w550 w555 w563 w568]
                tunnel: [w482 w483 w491 w496 w501 w506 w511 w516 w521 w527 w533 w539 w544 w549 w554 w562 w567] -> w479
                tunnel: w475 -> [_ w486 w490 w495 w500 w505 w510 w515 w520 w526 w532 w538 w543 w548 w553 w561 w566]
                tunnel: [TRUE _ _ _ _ _ _ _ _ _ _ _ _ _ _ _ _] -> w478
                frame "Stop", Default {
                }
                frame "Stop File Write" {
                  n171 = Variant To Data(error in=w487, type=FALSE, Variant=w486) -> (data=→"Stop File Write":bool, error out=w483:errorcluster)
                }
                frame "V1" {
                  n172 = Variant To Data(error in=w492, type=FALSE, Variant=w490) -> (data=w488:bool, error out=w491:errorcluster)
                  "V1" <- w488
                  n173 = shared-variable "NI-cRIO9022-019C2C95\\Mod6\\DO0"(w488) -> ()  [unwired: 1 in, 1 out]
                }
                frame "V2" {
                  n174 = Variant To Data(error in=w497, type=FALSE, Variant=w495) -> (data=w493:bool, error out=w496:errorcluster)
                  "V2" <- w493
                  n175 = shared-variable "NI-cRIO9022-019C2C95\\Mod6\\DO1"(w493) -> ()  [unwired: 1 in, 1 out]
                }
                frame "V3" {
                  n176 = Variant To Data(error in=w502, type=FALSE, Variant=w500) -> (data=w498:bool, error out=w501:errorcluster)
                  "V3" <- w498
                  n177 = shared-variable "NI-cRIO9022-019C2C95\\Mod6\\DO2"(w498) -> ()  [unwired: 1 in, 1 out]
                }
                frame "V4" {
                  n178 = Variant To Data(error in=w507, type=FALSE, Variant=w505) -> (data=w503:bool, error out=w506:errorcluster)
                  "V4" <- w503
                  n179 = shared-variable "NI-cRIO9022-019C2C95\\Mod6\\DO3"(w503) -> ()  [unwired: 1 in, 1 out]
                }
                frame "V10" {
                  n180 = Variant To Data(error in=w512, type=FALSE, Variant=w510) -> (data=w508:bool, error out=w511:errorcluster)
                  "V10" <- w508
                  n181 = shared-variable "NI-cRIO9022-019C2C95\\Mod7\\DO0"(w508) -> ()  [unwired: 1 in, 1 out]
                }
                frame "V11" {
                  n182 = Variant To Data(error in=w517, type=FALSE, Variant=w515) -> (data=w513:bool, error out=w516:errorcluster)
                  "V11" <- w513
                  n183 = shared-variable "NI-cRIO9022-019C2C95\\Mod7\\DO1"(w513) -> ()  [unwired: 1 in, 1 out]
                }
                frame "V12" {
                  n184 = Variant To Data(error in=w522, type=FALSE, Variant=w520) -> (data=w518:bool, error out=w521:errorcluster)
                  "V12" <- w518
                  n185 = shared-variable "NI-cRIO9022-019C2C95\\Mod7\\DO2"(w518) -> ()  [unwired: 1 in, 1 out]
                }
                frame "No_Flow" {
                  w523 = FALSE
                  n186 = Variant To Data(error in=w528, type=FALSE, Variant=w526) -> (data=→"FLOW ALL OFF":bool, error out=w527:errorcluster)
                  n187 = local write "LOW FLOW MASTER SWITCH"(w523) -> ()
                  n188 = local write "HIGH FLOW MASTER SWITCH"(w523) -> ()
                }
                frame "High_Flow" {
                  w529 = FALSE
                  n189 = Variant To Data(error in=w534, type=FALSE, Variant=w532) -> (data=→"HIGH FLOW MASTER SWITCH":bool, error out=w533:errorcluster)
                  n190 = local write "LOW FLOW MASTER SWITCH"(w529) -> ()
                  n191 = local write "FLOW ALL OFF"(w529) -> ()
                }
                frame "Low_Flow" {
                  w535 = FALSE
                  n192 = Variant To Data(error in=w540, type=FALSE, Variant=w538) -> (data=→"LOW FLOW MASTER SWITCH":bool, error out=w539:errorcluster)
                  n193 = local write "HIGH FLOW MASTER SWITCH"(w535) -> ()
                  n194 = local write "FLOW ALL OFF"(w535) -> ()
                }
                frame "MFC_1" {
                  n195 = Variant To Data(error in=w545, type=0.0, Variant=w543) -> (data=w541:dbl, error out=w544:errorcluster)
                  n196 = local write "MFC_1 SLPM set value"(w541) -> ()
                }
                frame "FGGA_restart" {
                  n197 = Variant To Data(error in=w550, type=FALSE, Variant=w548) -> (data=→"FGGA restart":bool, error out=w549:errorcluster)
                }
                frame "UDP Time Offset" {
                  n198 = Variant To Data(error in=w555, type=0, Variant=w553) -> (data=→"UDP Time Stamp Offset":i32, error out=w554:errorcluster)
                }
                frame "FGGA_pump" {
                  n199 = Variant To Data(error in=w563, type=FALSE, Variant=w561) -> (data=w558:bool, error out=w562:errorcluster)
                  "FGGA Pump" <- w558
                  n200 = Select(t=1.4 ("f"), s=w558, f=0.0 ("t")) -> (s? t:f=w559:dbl)
                  n201 = shared-variable "NI-cRIO9022-019C2C95\\Mod5\\AO0"(w559) -> ()  [unwired: 1 in, 1 out]
                }
                frame "Flight Number" {
                  n202 = Variant To Data(error in=w568, type="", Variant=w566) -> (data=→"Flight Number":string, error out=w567:errorcluster)
                }
              }
            }
            frame True {
            }
          }
          n203 = node-c288() -> ()  [unwired: 1 in, 1 out]
        }
        n204 = node-c288(w452) -> ()  [unwired: 1 out]
        n205 = Destroy Stream Endpoint(8:w456, 11:w455) -> (0:→"error out 2":errorcluster)
      }
      n206 = while {
        stop <- FALSE stop-if-true
        # "Emergency shutdown on the valves when connection to the client drops"
        n207 = shared-variable ".\\Global Shared Variables.lvlib\\Disconnect_WatchDog"() -> (w432:bool)  [unwired: 1 in, 1 out]
        n208 = Wait (ms)(milliseconds to wait=u32 1000) -> ()  [unwired: 1 out]
        n209 = case shown="True" w432 {
          frame False {
          }
          frame True {
            w439 = FALSE
            n210 = local read "HIGH FLOW MASTER SWITCH"() -> (w436:bool)
            n211 = local read "LOW FLOW MASTER SWITCH"() -> (w437:bool)
            n212 = local read "FLOW ALL OFF"() -> (w435:bool)
            n213 = case shown="True" w435 {
              frame False {
              }
              frame True {
                # "Disable eV10, 11& 12 & FGGA pump"
                n214 = flat-sequence {
                  frame #0 {
                    n215 = shared-variable "NI-cRIO9022-019C2C95\\Mod5\\AO0"(0.0) -> ()  [unwired: 1 in, 1 out]
                  }
                  frame #1 {
                    n216 = shared-variable "NI-cRIO9022-019C2C95\\Mod7\\DO1"(FALSE) -> ()  [unwired: 1 in, 1 out]
                  }
                  frame #2 {
                    n217 = shared-variable "NI-cRIO9022-019C2C95\\Mod7\\DO0"(FALSE) -> ()  [unwired: 1 in, 1 out]
                  }
                  frame #3 {
                    n218 = shared-variable "NI-cRIO9022-019C2C95\\Mod7\\DO2"(FALSE) -> ()  [unwired: 1 in, 1 out]
                  }
                }
              }
            }
            n219 = shared-variable "NI-cRIO9022-019C2C95\\Mod6\\DO1"(w439) -> ()  [unwired: 1 in, 1 out]
            n220 = case shown="True" w436 {
              frame False {
              }
              frame True {
                # "Disable FGGA pump & eV11, Enable eV10 & 12"
                n221 = flat-sequence {
                  frame #0 {
                    n222 = shared-variable "NI-cRIO9022-019C2C95\\Mod5\\AO0"(0.0) -> ()  [unwired: 1 in, 1 out]
                  }
                  frame #1 {
                    n223 = shared-variable "NI-cRIO9022-019C2C95\\Mod7\\DO1"(FALSE) -> ()  [unwired: 1 in, 1 out]
                  }
                  frame #2 {
                    n224 = shared-variable "NI-cRIO9022-019C2C95\\Mod7\\DO0"(TRUE) -> ()  [unwired: 1 in, 1 out]
                  }
                  frame #3 {
                    n225 = shared-variable "NI-cRIO9022-019C2C95\\Mod7\\DO2"(TRUE) -> ()  [unwired: 1 in, 1 out]
                  }
                }
              }
            }
            n226 = shared-variable "NI-cRIO9022-019C2C95\\Mod6\\DO3"(w439) -> ()  [unwired: 1 in, 1 out]
            n227 = shared-variable "NI-cRIO9022-019C2C95\\Mod6\\DO0"(w439) -> ()  [unwired: 1 in, 1 out]
            n228 = shared-variable "NI-cRIO9022-019C2C95\\Mod6\\DO2"(w439) -> ()  [unwired: 1 in, 1 out]
            n229 = case shown="True" w437 {
              frame False {
              }
              frame True {
                # "Disable eV10 & eV12, Enable eV11 & FGGA pump"
                n230 = flat-sequence {
                  frame #0 {
                    n231 = shared-variable "NI-cRIO9022-019C2C95\\Mod7\\DO0"(FALSE) -> ()  [unwired: 1 in, 1 out]
                  }
                  frame #1 {
                    n232 = shared-variable "NI-cRIO9022-019C2C95\\Mod7\\DO2"(FALSE) -> ()  [unwired: 1 in, 1 out]
                  }
                  frame #2 {
                    n233 = shared-variable "NI-cRIO9022-019C2C95\\Mod7\\DO1"(TRUE) -> ()  [unwired: 1 in, 1 out]
                  }
                  frame #3 {
                    n234 = shared-variable "NI-cRIO9022-019C2C95\\Mod5\\AO0"(1.4) -> ()  [unwired: 1 in, 1 out]
                  }
                }
              }
            }
            n235 = local write "MFC_1 SLPM set value"(0.0 ("MFC_1 SLPM set value")) -> ()
          }
        }
      }
      n236 = while {
        tunnel: w37 -> [w139]
        tunnel: w36 -> [w138]
        stop <- w140 stop-if-true
        # "Must Delay to avoid 100% CPU"
        # "Broadcast FGGA UDP Data"
        n237 = call-poly <vilib>:"UDP Multicast Open.vi"("time-to-live (1)"=u16 5, "port"=u16 10000) -> ("error out"=w147:errorcluster, "connection ID"=w148:refnum<k16>)  [unwired: 8 in]
        n238 = node-c288() -> (w150:T1)  [unwired: 4 in]
        n239 = timed-loop {
          tunnel: w148 -> [w171]
          tunnel: w147 -> [w170]
          timing: w150 -> [_]
          timing-out: [_] -> w149
          shift-right: [w159] -> _
          shift-left: FALSE -> [w162]
          tunnel: [w158] -> w142
          tunnel: [w156] -> w141
          tunnel: [w154] -> w140
          tunnel: w139 -> [w152]
          tunnel: w138 -> [w151]
          stop <- w155 stop-if-true
          # "UDP Broadcast loop"
          n240 = node-c288() -> ()  [unwired: 1 in, 1 out]
          n241 = local read "Flight Number"() -> (w153:string)
          n242 = feedback-in #2(w153) -> ()
          n243 = feedback #2() -> (w164:string)  [unwired: 1 in]
          n244 = Not Equal?(x=w153, y=w164) -> (x != y?=w163:bool)
          n245 = String To IP(1:"239.1.4.6" ("name")) -> (0:w168:u32)
          n246 = flat-sequence {
            tunnel: w168 -> [w178]
            tunnel: w170 -> [w179]
            tunnel: w171 -> [w180]
            tunnel: [w180] -> w167
            tunnel: [w179] -> w166
            tunnel: [w178] -> w165
            tunnel: w163 -> [w177]
            tunnel: u16 50001 ("port or service name") -> [w191]
            tunnel: w167 -> [w190]
            tunnel: w166 -> [w189]
            tunnel: w165 -> [w188]
            tunnel: [w187] -> w158
            tunnel: [w186] -> w156
            tunnel: w152 -> [w184]
            tunnel: w151 -> [w183]
            frame #0 {
              n247 = feedback #3(u32 0) -> (w174:u32)
              n248 = case shown="False" w177 {
                tunnel: w174 -> [w181 _]
                tunnel: [w181 u32 0] -> w173
                frame False {
                }
                frame True {
                }
              }
              "UDP_Pack_num" <- w173
              n249 = Increment(x=w173) -> (x+1=w175:u32)
              n250 = feedback-in #3(w175) -> ()
            }
            frame #1 {
              n251 = Dequeue Element(queue=w184, error in (no error)=w183) -> (element=w185:string)  [unwired: 1 in, 3 out]
              n252 = UDP Write(address=w188, port or service name=w191, connection ID=w190, data in=w185, 8:w189) -> (error out=w186:errorcluster, 3:w187:refnum<k16>)  [unwired: 1 in]
            }
          }
          n253 = Select(t=FALSE, s=w162, f=TRUE) -> (s? t:f=w159:bool)
          "UDP_Out Status" <- w159
          n254 = local read "stop"() -> (w154:bool)
          n255 = node-c288() -> ()  [unwired: 1 in, 1 out]
          n256 = Unbundle(w156) -> ("status"=w157:bool)  [unwired: 2 out]
          n257 = Compound Arithmetic op=OR(w157, w154) -> (w155:bool)
        }
        n258 = node-c288(w149) -> ()  [unwired: 1 out]
        n259 = UDP Close(connection ID=w142, 8:w141) -> (error out=→"UDP_Out_Error Out":errorcluster)  [unwired: 1 out]
        n260 = Wait (ms)(milliseconds to wait=u32 1000) -> ()  [unwired: 1 out]
      }
      n261 = node-c288(w23) -> ()  [unwired: 1 out]
      n262 = while {
        tunnel: w33 -> [w97]
        tunnel: w32 -> [w96]
        stop <- w100 stop-if-true
        # "Must Delay to avoid 100% CPU"
        # "TCP Loop writing to FISH Tank"
        n263 = TCP Open Connection(address="192.168.101.110", remote port or service name=u16 3502) -> (connection ID=w103:refnum<k5>, error out=w98:errorcluster)  [unwired: 3 in]
        n264 = case shown="No Error" w98 {
          selector: w98 -> [w108 w135]
          tunnel: w103 -> [w113 w136]
          tunnel: [w112 w136] -> w102
          tunnel: [w111 w135] -> w101
          tunnel: [w110 w134] -> w100
          tunnel: w97 -> [w107 _]
          tunnel: w96 -> [w106 _]
          frame No Error {
            n265 = node-c288() -> (w115:T1)  [unwired: 4 in]
            n266 = timed-loop {
              tunnel: w113 -> [w129]
              tunnel: w108 -> [w128]
              tunnel: [w127] -> w112
              tunnel: [w126] -> w111
              tunnel: [w118] -> w110
              shift-right: [w120] -> _
              shift-left: FALSE -> [w123]
              timing: w115 -> [_]
              timing-out: [_] -> w114
              tunnel: w107 -> [w117]
              tunnel: w106 -> [w116]
              stop <- w124 stop-if-true
              n267 = node-c288() -> ()  [unwired: 1 in, 1 out]
              n268 = Dequeue Element(queue=w117, error in (no error)=w116) -> (element=w119:string)  [unwired: 1 in, 3 out]
              n269 = Select(t=FALSE, s=w123, f=TRUE) -> (s? t:f=w120:bool)
              "TCP packet\nSend To FISH" <- w120
              n270 = TCP Write(connection ID=w129, data in=w119, error in (no error)=w128) -> (connection ID out=w127:refnum<k5>, error out=w126:errorcluster)  [unwired: 1 in, 1 out]
              n271 = local read "stop"() -> (w118:bool)
              n272 = Unbundle(w126) -> ("status"=w125:bool)  [unwired: 2 out]
              n273 = node-c288() -> ()  [unwired: 1 in, 1 out]
              n274 = Compound Arithmetic op=OR(w125, w118) -> (w124:bool)
            }
            n275 = node-c288(w114) -> ()  [unwired: 1 out]
          }
          frame Error {
            n276 = local read "stop"() -> (w134:bool)
          }
        }
        n277 = TCP Close Connection(connection ID=w102, error in (no error)=w101) -> (error out=→"FISH TCP Error Out":errorcluster)  [unwired: 1 in, 1 out]
        n278 = Wait (ms)(milliseconds to wait=u32 1000) -> ()  [unwired: 1 out]
      }
      n279 = while {
        tunnel: w35 -> [w392]
        tunnel: w34 -> [w391]
        stop <- w395 stop-if-true
        # "Must Delay to avoid 100% CPU"
        # "TCP Loop writing to SEPTIC Tank"
        n280 = TCP Open Connection(address="192.168.101.108", remote port or service name=u16 3502) -> (connection ID=w398:refnum<k5>, error out=w393:errorcluster)  [unwired: 3 in]
        n281 = case shown="No Error" w393 {
          selector: w393 -> [w403 w430]
          tunnel: w398 -> [w408 w431]
          tunnel: [w407 w431] -> w397
          tunnel: [w406 w430] -> w396
          tunnel: [w405 w429] -> w395
          tunnel: w392 -> [w402 _]
          tunnel: w391 -> [w401 _]
          frame No Error {
            n282 = node-c288() -> (w410:T1)  [unwired: 4 in]
            n283 = timed-loop {
              tunnel: w408 -> [w424]
              tunnel: w403 -> [w423]
              tunnel: [w422] -> w407
              tunnel: [w421] -> w406
              tunnel: [w413] -> w405
              shift-right: [w415] -> _
              shift-left: FALSE -> [w418]
              timing: w410 -> [_]
              timing-out: [_] -> w409
              tunnel: w402 -> [w412]
              tunnel: w401 -> [w411]
              stop <- w419 stop-if-true
              n284 = node-c288() -> ()  [unwired: 1 in, 1 out]
              n285 = Dequeue Element(queue=w412, error in (no error)=w411) -> (element=w414:string)  [unwired: 1 in, 3 out]
              n286 = Select(t=FALSE, s=w418, f=TRUE) -> (s? t:f=w415:bool)
              "TCP packet\nSend To SEPTIC" <- w415
              n287 = TCP Write(connection ID=w424, data in=w414, error in (no error)=w423) -> (connection ID out=w422:refnum<k5>, error out=w421:errorcluster)  [unwired: 1 in, 1 out]
              n288 = local read "stop"() -> (w413:bool)
              n289 = Unbundle(w421) -> ("status"=w420:bool)  [unwired: 2 out]
              n290 = node-c288() -> ()  [unwired: 1 in, 1 out]
              n291 = Compound Arithmetic op=OR(w420, w413) -> (w419:bool)
            }
            n292 = node-c288(w409) -> ()  [unwired: 1 out]
          }
          frame Error {
            n293 = local read "stop"() -> (w429:bool)
          }
        }
        n294 = TCP Close Connection(connection ID=w397, error in (no error)=w396) -> (error out=→"SEPTIC TCP Error Out":errorcluster)  [unwired: 1 in, 1 out]
        n295 = Wait (ms)(milliseconds to wait=u32 1000) -> ()  [unwired: 1 out]
      }
    }
    frame Error {
    }
  }
  n296 = VISA Close(VISA resource name=w17, error in (no error)=w18) -> (error out=→"Serial error out":errorcluster)
